vi "WPI_SolenoidOpenSingle.vi"(8 "error in (no error)":errorcluster, 10 "Solenoid Channel":T1, 11 "Pneumatics Control Module (0)":u8) -> (0 "error out":errorcluster, 3 "SolenoidDevRef":T2={"DevStatus"={"status"=FALSE, "code"=0, "source"=""}, "Pneumatics Control Module"=0, "Forward Solenoid Channel"=enum."Invalid", "Reverse Solenoid Channel"=enum."Invalid"})   [LabVIEW 2017]
doc: "Opens a reference to the solenoid you specify. You must open a reference before using any other VIs on this palette.\n\nThis software is licensed. Open the labview\\readme\\WPI Robotics Library Open Source License.txt file for more information."
uses:
  <vilib>/Rock Robotics/WPI/Solenoid/WPI_SolenoidDevRef.ctl
  <vilib>/Rock Robotics/WPI/Solenoid/WPI_SolenoidChannel.ctl
  <vilib>/Rock Robotics/WPI/Solenoid/WPI_SolenoidCacheOp.ctl
  <vilib>/Rock Robotics/SystemInterfaces/NetworkCommunication/NetComm_UsageReport_ResourceType.ctl
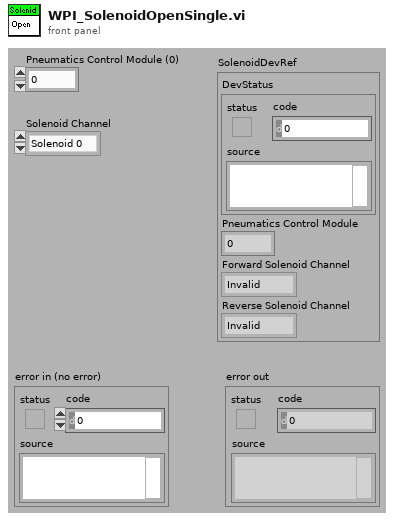
[diagram p1: front panel]
types:
  T1 = typedef "WPI_SolenoidChannel.ctl" = enum8{"Solenoid 0", "Solenoid 1", "Solenoid 2", "Solenoid 3", "Solenoid 4", "Solenoid 5", "Solenoid 6", "Solenoid 7", "Invalid"}
  T2 = typedef "WPI_SolenoidDevRef.ctl" = cluster{"DevStatus":errorcluster, "Pneumatics Control Module":u8, "Forward Solenoid Channel":T1, "Reverse Solenoid Channel":T1}
  T3 = typedef "NetComm_UsageReport_ResourceType.ctl" = enum8{"Controller", "Module", "Language", "CANPlugin", "Accelerometer", "ADXL345", "AnalogChannel", "AnalogTrigger", "AnalogTriggerOutput", "CANJaguar", "Compressor", "Counter", "Dashboard", "DigitalInput", "DigitalOutput", "DriverStationCIO", "DriverStationEIO", "DriverStationLCD", "Encoder", "GearTooth", "Gyro", "I2C", "Framework", "Jaguar", "Joystick", "Kinect", "KinectStick", "PIDController", "Preferences", "PWM", "Relay", "RobotDrive", "SerialPort", "Servo", "Solenoid", "SPI", "Task", "Ultrasonic", "Victor", "Button", "Command", "AxisCamera", "PCVideoServer", "SmartDashboard", "Talon", "HiTechnicColorSensor", "HiTechnicAccel", "HiTechnicCompass", "SRF08", "AnalogOutput", "Victor SP", "Talon SRX", "CAN Talon SRX", "ADXL362 Accel", "ADXRS450 Gyro", "Rev SPARK", "Mindsensors SD540", "Digital Filter", "ADIS16448", "PDP", "PCM", "PigeonIMU", "Nidec Brushless", "CTRE CANifier", "CTRE Future 0", "CTRE Future 1", "CTRE Future 2", "CTRE Future 3", "CTRE Future 4", "CTRE Future 5", "CTRE Future 6"}
  T4 = typedef "WPI_SolenoidCacheOp.ctl" = enum16{"Acquire", "Release", "Status"}
  T5 = typedef "WPI_CompressorDevRef.ctl" = cluster{"DevStatus":errorcluster, "Pneumatics Control Module":u8}
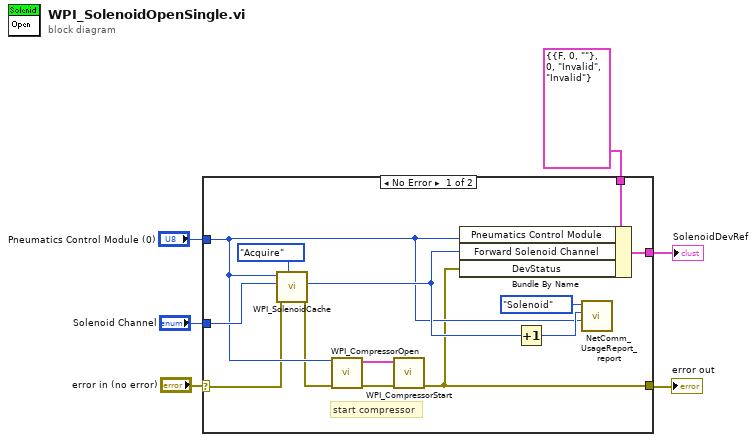
[diagram p0: block diagram]
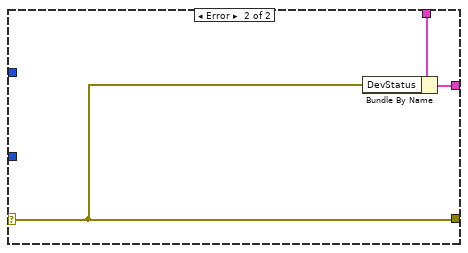
[diagram p2: hidden frame]
diagram:
  n1 = case shown="No Error" "error in (no error)" {
    selector: "error in (no error)" -> [w8 w20]
    tunnel: [w9 w20] -> w5
    tunnel: [w18 w22] -> w3
    tunnel: "Solenoid Channel" -> [w16 _]
    tunnel: "Pneumatics Control Module (0)" -> [w10 _]
    tunnel: T2 {"DevStatus"={"status"=FALSE, "code"=0, "source"=""}, "Pneumatics Control Module"=0, "Forward Solenoid Channel"=enum."Invalid", "Reverse Solenoid Channel"=enum."Invalid"} ("SolenoidDevRef") -> [w19 w21]
    frame No Error {
      # "start compressor"
      n2 = call <vilib>:"WPI_SolenoidCache.vi"("AllocatedSolenoidOp"=WPI_SolenoidCacheOp."Acquire", "error in (no error)"=w8, "SolenoidChannel"=w16, "Pneumatics Control Module"=w10) -> ("error out"=w7:errorcluster, "AllocatedSolenoidChannel"=w14:T1)  [unwired: 1 in, 5 out]
      n3 = call <vilib>:"WPI_CompressorOpen.vi"("Pneumatics Control Module (0)"=w10, "error in (no error)"=w7) -> ("CompressorDevRef"=w11:T5, "error out"=w12:errorcluster)  [unwired: 12 in]
      n4 = call <vilib>:"WPI_CompressorStart.vi"("error in (no error)"=w12, "CompressorDevRef"=w11) -> ("error out"=w9:errorcluster)  [unwired: 8 in, 1 out]
      n5 = Bundle By Name(cluster=w19, "Pneumatics Control Module"=w10, "Forward Solenoid Channel"=w14, "DevStatus"=w9) -> (w18:T2)
      n6 = Increment(x=w14) -> (x+1=w13:T1)
      n7 = call <vilib>:"NetComm_UsageReport_report.vi"("Context"=w10, "Instance Number"=w13, "Resource Type"=NetComm_UsageReport_ResourceType."Solenoid") -> ()  [unwired: 9 in]
    }
    frame Error {
      n8 = Bundle By Name(cluster=w21, "DevStatus"=w20) -> (w22:T2)
    }
  }
  "SolenoidDevRef" <- w3
  "error out" <- w5
